vi "CS4_status.vi"(0 "address string":string, 1 "error in":errorcluster) -> (2 "RATE (Range 1) (T/min)":dbl, 3 "RATE (Range 2) (T/min)":dbl, 4 "RATE (Range 3) (T/min)":dbl, 5 "Sweep mode":string, 6 "Real Field":string, 7 "Sweep Set Point (Low)":string, 8 "Sweep Set Point (High)":string, 9 "Arrive":bool, 10 "error out":errorcluster)   [LabVIEW 2012]
panel:
  out "RATE (Range 3)":string
  out "RATE (Range 2)":string
  out "RATE (Range 1)":string
  out "Heater on?":bool
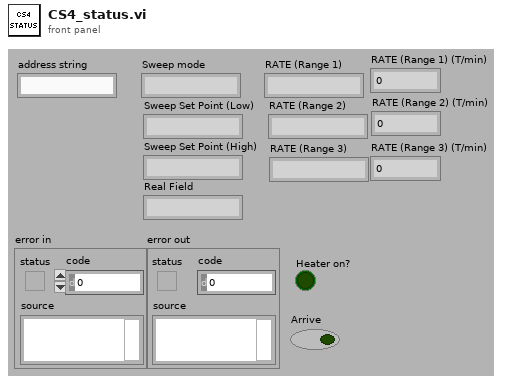
[diagram p1: front panel]
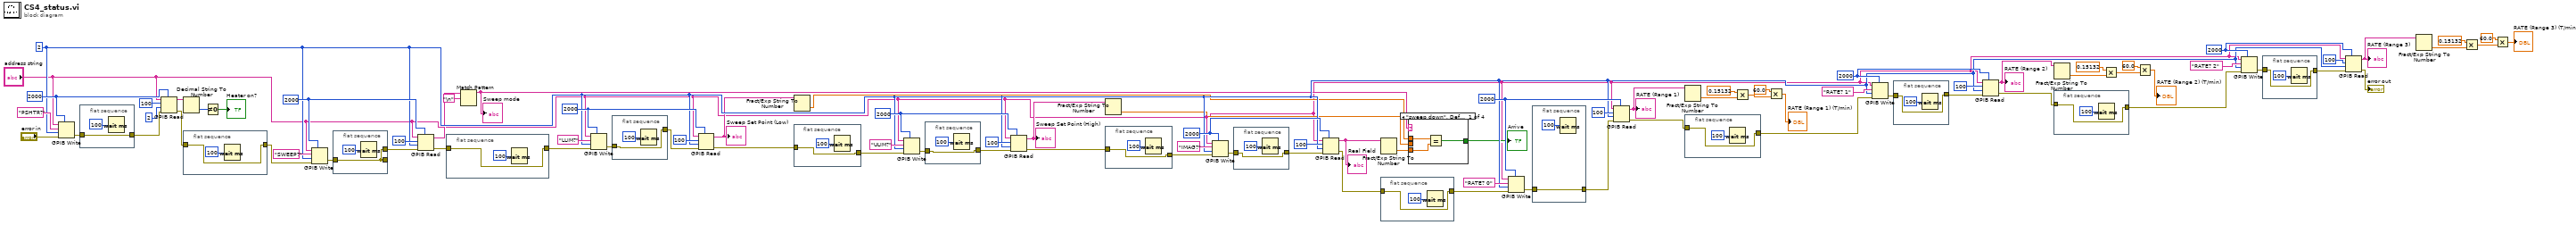
[diagram p0: block diagram]
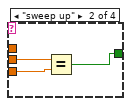
[diagram p2: hidden frame]
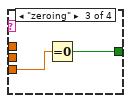
[diagram p3: hidden frame]
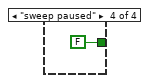
[diagram p4: hidden frame]
diagram:
  w64 = 2000 ("timeout ms (488.2 global)")
  w66 = 2000 ("timeout ms (488.2 global)")
  w67 = 2000 ("timeout ms (488.2 global)")
  w72 = 2000 ("timeout ms (488.2 global)")
  w74 = 2000 ("timeout ms (488.2 global)")
  w77 = 2000 ("timeout ms (488.2 global)")
  w78 = 2000 ("timeout ms (488.2 global)")
  w87 = 2000 ("timeout ms (488.2 global)")
  w61 = i16 2 ("mode (0)")
  n1 = GPIB Write(0:"address string", 1:"PSHTR?" ("data"), 2:w61, 3:"error in", 4:w87) -> (6:w17:errorcluster)  [unwired: 1 out]
  n2 = flat-sequence {
    tunnel: w17 -> [w91]
    tunnel: [w91] -> w16
    frame #0 {
      n3 = Wait (ms)(milliseconds to wait=u32 100) -> ()  [unwired: 1 out]
    }
  }
  n4 = GPIB Read(0:"address string", 1:100 ("byte count"), 2:i16 2 ("mode (0)"), 3:w16, 4:w87) -> (5:w85:string, 7:w32:errorcluster)  [unwired: 1 out]
  n5 = Decimal String To Number(string=w85) -> (number=w84:i32)  [unwired: 2 in, 1 out]
  n6 = flat-sequence {
    tunnel: w32 -> [w93]
    tunnel: [w93] -> w31
    frame #0 {
      n7 = Wait (ms)(milliseconds to wait=u32 100) -> ()  [unwired: 1 out]
    }
  }
  n8 = Not Equal To 0?(x=w84) -> (x != 0?=→"Heater on?":bool)
  n9 = GPIB Write(0:"address string", 1:"SWEEP?" ("data"), 2:w61, 3:w31, 4:w78) -> (6:w15:errorcluster)  [unwired: 1 out]
  n10 = flat-sequence {
    tunnel: w15 -> [w95]
    tunnel: [w95] -> _
    tunnel: [w95] -> w14
    frame #0 {
      n11 = Wait (ms)(milliseconds to wait=u32 100) -> ()  [unwired: 1 out]
    }
  }
  n12 = GPIB Read(0:"address string", 1:100 ("byte count"), 2:w61, 3:w14, 4:w78) -> (5:w53:string, 7:w30:errorcluster)  [unwired: 1 out]
  n13 = flat-sequence {
    tunnel: w30 -> [w97]
    tunnel: [w97] -> w29
    frame #0 {
      n14 = Wait (ms)(milliseconds to wait=u32 100) -> ()  [unwired: 1 out]
    }
  }
  n15 = Match Pattern(string=w53, regular expression="\n") -> (before substring=w52:string)  [unwired: 1 in, 3 out]
  "Sweep mode" <- w52
  n16 = GPIB Write(0:"address string", 1:"LLIM?" ("data"), 2:w61, 3:w29, 4:w77) -> (6:w12:errorcluster)  [unwired: 1 out]
  n17 = flat-sequence {
    tunnel: w12 -> [w99]
    tunnel: [w99] -> w11
    frame #0 {
      n18 = Wait (ms)(milliseconds to wait=u32 100) -> ()  [unwired: 1 out]
    }
  }
  n19 = GPIB Read(0:"address string", 1:100 ("byte count"), 2:w61, 3:w11, 4:w77) -> (5:w58:string, 7:w28:errorcluster)  [unwired: 1 out]
  "Sweep Set Point (Low)" <- w58
  n20 = Fract/Exp String To Number(string=w58) -> (number=w56:dbl)  [unwired: 3 in, 1 out]
  n21 = flat-sequence {
    tunnel: w28 -> [w101]
    tunnel: [w101] -> w27
    frame #0 {
      n22 = Wait (ms)(milliseconds to wait=u32 100) -> ()  [unwired: 1 out]
    }
  }
  n23 = GPIB Write(0:"address string", 1:"ULIM?" ("data"), 2:w61, 3:w27, 4:w74) -> (6:w10:errorcluster)  [unwired: 1 out]
  n24 = flat-sequence {
    tunnel: w10 -> [w103]
    tunnel: [w103] -> w9
    frame #0 {
      n25 = Wait (ms)(milliseconds to wait=u32 100) -> ()  [unwired: 1 out]
    }
  }
  n26 = GPIB Read(0:"address string", 1:100 ("byte count"), 2:w61, 3:w9, 4:w74) -> (5:w57:string, 7:w26:errorcluster)  [unwired: 1 out]
  "Sweep Set Point (High)" <- w57
  n27 = Fract/Exp String To Number(string=w57) -> (number=w55:dbl)  [unwired: 3 in, 1 out]
  n28 = flat-sequence {
    tunnel: w26 -> [w105]
    tunnel: [w105] -> w25
    frame #0 {
      n29 = Wait (ms)(milliseconds to wait=u32 100) -> ()  [unwired: 1 out]
    }
  }
  n30 = GPIB Write(0:"address string", 1:"IMAG?" ("data"), 2:w61, 3:w25, 4:w72) -> (6:w8:errorcluster)  [unwired: 1 out]
  n31 = flat-sequence {
    tunnel: w8 -> [w107]
    tunnel: [w107] -> w7
    frame #0 {
      n32 = Wait (ms)(milliseconds to wait=u32 100) -> ()  [unwired: 1 out]
    }
  }
  n33 = GPIB Read(0:"address string", 1:100 ("byte count"), 2:w61, 3:w7, 4:w72) -> (5:w60:string, 7:w24:errorcluster)  [unwired: 1 out]
  "Real Field" <- w60
  n34 = Fract/Exp String To Number(string=w60) -> (number=w59:dbl)  [unwired: 3 in, 1 out]
  n35 = flat-sequence {
    tunnel: w24 -> [w109]
    tunnel: [w109] -> w23
    frame #0 {
      n36 = Wait (ms)(milliseconds to wait=u32 100) -> ()  [unwired: 1 out]
    }
  }
  n37 = case shown="\"sweep down\", Default" w52 {
    tunnel: w59 -> [w112 w116 w118 _]
    tunnel: w56 -> [w113 _ _ _]
    tunnel: w55 -> [_ w115 _ _]
    tunnel: [w111 w114 w117 FALSE] -> w54
    frame "sweep down", Default {
      n38 = Equal?(x=w113, y=w112) -> (x = y?=w111:bool)
    }
    frame "sweep up" {
      n39 = Equal?(x=w115, y=w116) -> (x = y?=w114:bool)
    }
    frame "zeroing" {
      n40 = Equal To 0?(x=w118) -> (x = 0?=w117:bool)
    }
    frame "sweep paused" {
    }
  }
  "Arrive" <- w54
  n41 = GPIB Write(0:"address string", 1:"RATE? 0" ("data"), 2:w61, 3:w23, 4:w67) -> (6:w6:errorcluster)  [unwired: 1 out]
  n42 = flat-sequence {
    tunnel: w6 -> [w120]
    tunnel: [w120] -> w5
    frame #0 {
      n43 = Wait (ms)(milliseconds to wait=u32 100) -> ()  [unwired: 1 out]
    }
  }
  n44 = GPIB Read(0:"address string", 1:100 ("byte count"), 2:w61, 3:w5, 4:w67) -> (5:w50:string, 7:w22:errorcluster)  [unwired: 1 out]
  "RATE (Range 1)" <- w50
  n45 = Fract/Exp String To Number(string=w50) -> (number=w49:dbl)  [unwired: 3 in, 1 out]
  n46 = flat-sequence {
    tunnel: w22 -> [w122]
    tunnel: [w122] -> w21
    frame #0 {
      n47 = Wait (ms)(milliseconds to wait=u32 100) -> ()  [unwired: 1 out]
    }
  }
  n48 = Multiply(x=0.15132, y=w49) -> (x*y=w47:dbl)
  n49 = Multiply(x=60.0, y=w47) -> (x*y=→"RATE (Range 1) (T/min)":dbl)
  n50 = GPIB Write(0:"address string", 1:"RATE? 1" ("data"), 2:w61, 3:w21, 4:w66) -> (6:w4:errorcluster)  [unwired: 1 out]
  n51 = flat-sequence {
    tunnel: w4 -> [w124]
    tunnel: [w124] -> w3
    frame #0 {
      n52 = Wait (ms)(milliseconds to wait=u32 100) -> ()  [unwired: 1 out]
    }
  }
  n53 = GPIB Read(0:"address string", 1:100 ("byte count"), 2:w61, 3:w3, 4:w66) -> (5:w34:string, 7:w20:errorcluster)  [unwired: 1 out]
  "RATE (Range 2)" <- w34
  n54 = Fract/Exp String To Number(string=w34) -> (number=w44:dbl)  [unwired: 3 in, 1 out]
  n55 = flat-sequence {
    tunnel: w20 -> [w126]
    tunnel: [w126] -> w19
    frame #0 {
      n56 = Wait (ms)(milliseconds to wait=u32 100) -> ()  [unwired: 1 out]
    }
  }
  n57 = Multiply(x=0.15132, y=w44) -> (x*y=w42:dbl)
  n58 = Multiply(x=60.0, y=w42) -> (x*y=→"RATE (Range 2) (T/min)":dbl)
  n59 = GPIB Write(0:"address string", 1:"RATE? 2" ("data"), 2:w61, 3:w19, 4:w64) -> (6:w2:errorcluster)  [unwired: 1 out]
  n60 = flat-sequence {
    tunnel: w2 -> [w128]
    tunnel: [w128] -> w1
    frame #0 {
      n61 = Wait (ms)(milliseconds to wait=u32 100) -> ()  [unwired: 1 out]
    }
  }
  n62 = GPIB Read(0:"address string", 1:100 ("byte count"), 2:w61, 3:w1, 4:w64) -> (5:w33:string, 7:→"error out":errorcluster)  [unwired: 1 out]
  "RATE (Range 3)" <- w33
  n63 = Fract/Exp String To Number(string=w33) -> (number=w39:dbl)  [unwired: 3 in, 1 out]
  n64 = Multiply(x=0.15132, y=w39) -> (x*y=w37:dbl)
  n65 = Multiply(x=60.0, y=w37) -> (x*y=→"RATE (Range 3) (T/min)":dbl)
